vi "Variant to JSON Text EXPERIMENT.vi"(6 "Pretty Print?":bool, 7 "enable LabVIEW extensions? (T)":bool=TRUE, 9 "error in (no error)":errorcluster, 11 "Variant":variant) -> (1 "error out":errorcluster, 3 "<JSON>":string)   [LabVIEW 2015, in "JSONtext.lvlib"]
doc: "Converts a LabVIEW datatype (<b>Variant</b>) into a JSON value. \n\nStrings or Arrays of strings marked with a leading \"<JSON>\" tag in their name (including inside clusters) are treated as already being valid JSON. Strings not marked as <JSON> are quoted and escaped as a JSON String. Note that JSONtext.lvlib functions that produce JSON have their outputs labelled \"<JSON>\", so that they may be used as inputs to other functions.\n\nTwo types of LabVIEW Clusters are supported: either with all named elements, which are converted to JSON Objects, or all unnamed elements (or elements just named \"<JSON>\"), which are converted to a JSON Array. Handling of mixed clusters with some named and some unnamed in undefined (currently, this VI will use the first element to determine whether to convert to an Object or Array)."
uses:
  JSONtext.lvlib
panel:
  out "Name of data in Variant":string
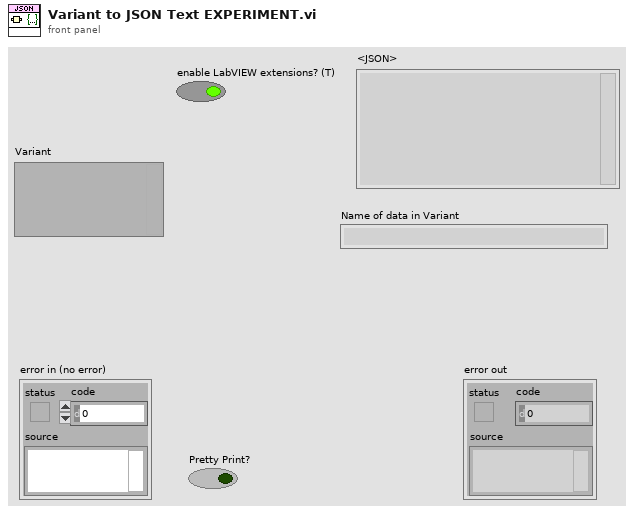
[diagram p1: front panel]
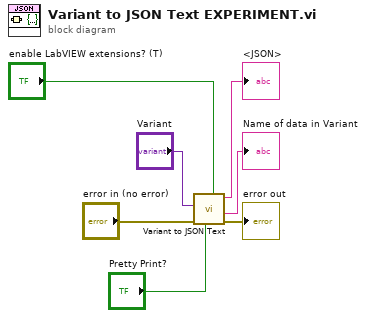
[diagram p0: block diagram]
diagram:
  n1 = call "Variant to JSON Text.vi"("enable LabVIEW extensions? (T)"="enable LabVIEW extensions? (T)", "Pretty Print?"="Pretty Print?", "error in (no error)"="error in (no error)", "Variant"="Variant") -> ("error out"=→"error out":errorcluster, "Name of data in Variant"=→"Name of data in Variant":string, "<JSON>"=→"<JSON>":string)  [unwired: 5 in]
